vi "CMD_FLEXREAD.vi"(6 "Gantry Class in":refnum<class "Gantry.lvclass">, 8 "error in (no error)":errorcluster, 10 "Arguments":string[](array[string]), 11 "gScript Interpreter in":refnum<class "gScript Interpreter.lvclass">) -> (0 "error out":errorcluster, 3 "gScript Interpreter out":refnum<class "gScript Interpreter.lvclass">, 4 "Gantry Class out":refnum<class "Gantry.lvclass">)   [LabVIEW 2017, in "gScript Interpreter.lvclass"]
uses:
  gScript Interpreter.lvclass
  Shared Components/Gantry Class/Gantry.lvclass
  Type Definitions/Memory Cell.ctl
  Type Definitions/Memory Cell Type Enum.ctl
  Shared Components/FlexWorktable/FlexWorktable.lvclass
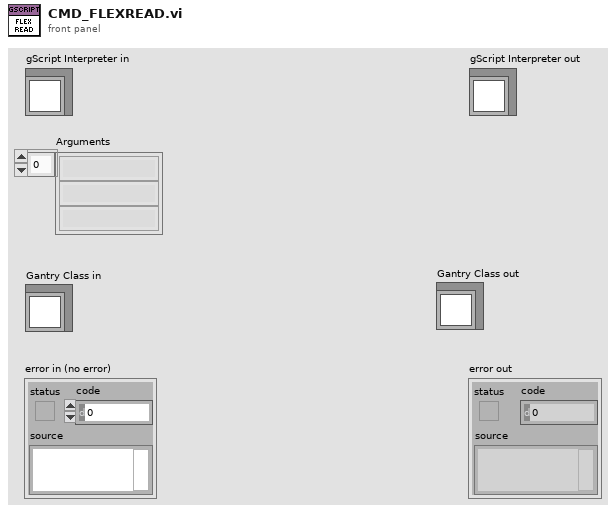
[diagram p1: front panel]
types:
  T1 = typedef "Memory Cell.ctl" = cluster{"type":T2, "x":dbl, "y":dbl, "z":dbl, "w":dbl}
  T2 = typedef "Memory Cell Type Enum.ctl" = enum16{"integer", "float", "vector", "rotation"}
  T3 = cluster{i32, dbl, string, bool, "Orient3d Class.lvclass":refnum<class "Orient3d.lvclass">, "Vec3d Class.lvclass":refnum<class "Vec3d.lvclass">}
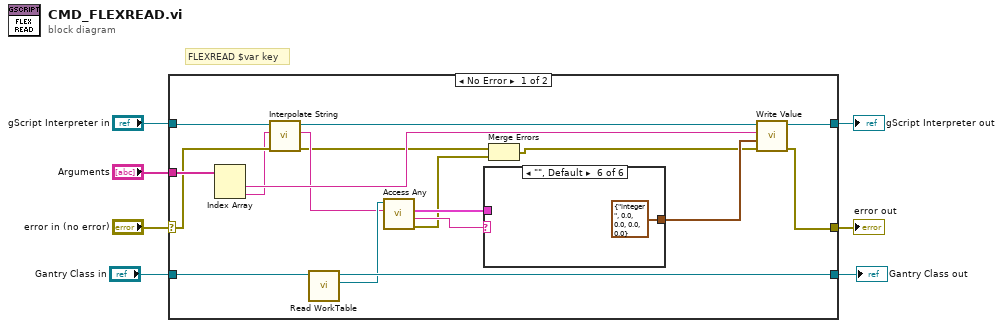
[diagram p0: block diagram]
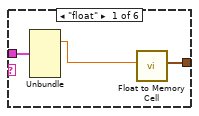
[diagram p2: hidden frame]
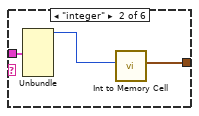
[diagram p3: hidden frame]
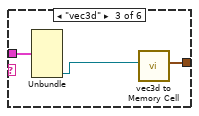
[diagram p4: hidden frame]
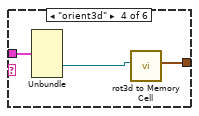
[diagram p5: hidden frame]
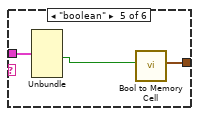
[diagram p6: hidden frame]
diagram:
  # "FLEXREAD $var key"
  n1 = case shown="No Error" "error in (no error)" {
    selector: "error in (no error)" -> [w20 w44]
    tunnel: [w23 w44] -> w6
    tunnel: [w22 w43] -> w4
    tunnel: "gScript Interpreter in" -> [w21 w43]
    tunnel: "Arguments" -> [w24 _]
    tunnel: "Gantry Class in" -> [w18 w42]
    tunnel: [w17 w42] -> w1
    frame No Error {
      n2 = Index Array(array=w24) -> (element #1=w25:string, element #2=w8:string)  [unwired: 2 in]
      n3 = call-dynamic "Interpolate String.vi"("error in (no error)"=w20, "Input String"=w8, "gScript Interpreter in"=w21) -> ("error out"=w11:errorcluster, "Output String"=w14:string, "gScript Interpreter out"=w16:refnum<class "gScript Interpreter.lvclass">)  [unwired: 6 in]
      n4 = call-dynamic "Read WorkTable.vi"("Gantry Class in"=w18) -> ("Worktable"=w15:refnum<class "FlexWorktable.lvclass">, "Gantry Class out"=w17:refnum<class "Gantry.lvclass">)  [unwired: 8 in, 1 out]
      n5 = call-dynamic "Access Any.vi"("Key"=w14, "FlexWorktable in"=w15) -> ("error out"=w10:errorcluster, "Type"=w13:string, "Items out"=w12:T3)  [unwired: 6 in, 1 out]
      n6 = case shown="\"\", Default" w13 {
        tunnel: [w28 w31 w34 w37 w39 T1 {"type"=enum."integer", "x"=0.0, "y"=0.0, "z"=0.0, "w"=0.0} ("Memory Cell")] -> w19
        tunnel: w12 -> [w27 w30 w33 w36 w40 _]
        frame "float" {
          n7 = Unbundle(w27) -> (w26:dbl)  [unwired: 5 out]
          n8 = call "Float to Memory Cell.vi"("Float in"=w26) -> ("Memory Cell"=w28:T1)  [unwired: 10 in]
        }
        frame "integer" {
          n9 = Unbundle(w30) -> (w29:i32)  [unwired: 5 out]
          n10 = call "Int to Memory Cell.vi"("Numeric"=w29) -> ("Memory Cell"=w31:T1)  [unwired: 10 in]
        }
        frame "vec3d" {
          n11 = Unbundle(w33) -> ("Vec3d Class.lvclass"=w32:refnum<class "Vec3d.lvclass">)  [unwired: 5 out]
          n12 = call "vec3d to Memory Cell.vi"("Vec3d in"=w32) -> ("Memory Cell"=w34:T1)  [unwired: 10 in]
        }
        frame "orient3d" {
          n13 = Unbundle(w36) -> ("Orient3d Class.lvclass"=w35:refnum<class "Orient3d.lvclass">)  [unwired: 5 out]
          n14 = call "rot3d to Memory Cell.vi"("Orient3d in"=w35) -> ("Memory Cell"=w37:T1)  [unwired: 10 in]
        }
        frame "boolean" {
          n15 = Unbundle(w40) -> (w38:bool)  [unwired: 5 out]
          n16 = call "Bool to Memory Cell.vi"("Boolean in"=w38) -> ("Memory Cell"=w39:T1)  [unwired: 10 in]
        }
        frame "", Default {
        }
      }
      n17 = Merge Errors(w11, w10) -> (w9:errorcluster)
      n18 = call-dynamic "Write Value.vi"("error in (no error)"=w9, "Value"=w19, "Address"=w25, "gScript Interpreter in"=w16) -> ("error out"=w23:errorcluster, "gScript Interpreter out"=w22:refnum<class "gScript Interpreter.lvclass">)  [unwired: 6 in]
    }
    frame Error {
    }
  }
  "error out" <- w6
  "gScript Interpreter out" <- w4
  "Gantry Class out" <- w1
